vi "DMM Read DC Voltage.vi"() -> ()   [LabVIEW 2011]
uses:
  <instrlib>/DMM4/DMM4.lvlib
panel:
  out "error out":errorcluster
  out "Measure Value":string
  in  "Stop":bool
  out "Boolean":bool
  in  "Detector Rate":u16(ring) items=["SLOW", "MID", "FAST"]
  in  "Manual Range":dbl format="%#.9e"
  in  "Enable Auto Range":bool=TRUE
  out "ID Return String":string
  in  "Configure RS232 Baud Rate":u32(ring)=115200 items=["9600"=9600, "19200"=19200, "38400"=38400, "57600"=57600, "115200"=115200]
  in  "VISA resource name":refnum<visa-resource-name>
  # "DMM Read DC Voltage"
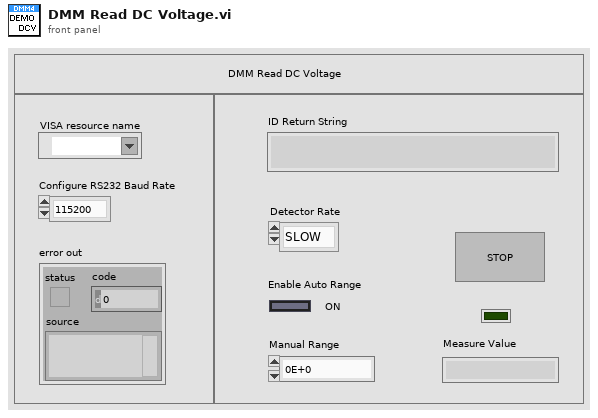
[diagram p1: front panel]
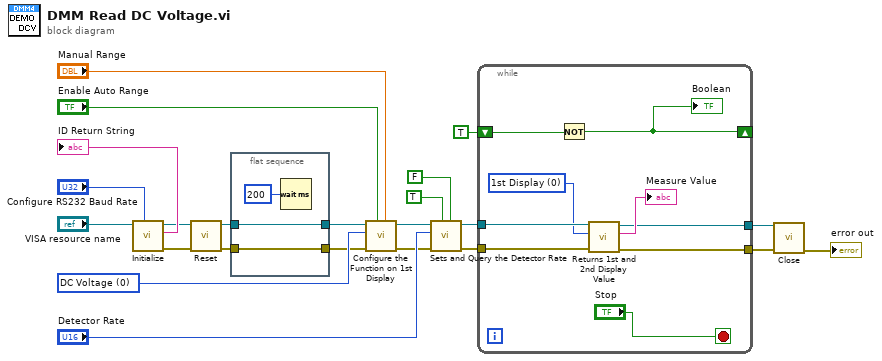
[diagram p0: block diagram]
diagram:
  w20 = u8 0 items=["DC Voltage", "AC Voltage", "DC+AC Voltage", "DC Current", "AC Current", "DC+AC Current", "2-Wire Resistance", "Frequency", "Period", "Continuity", "Diode", "Temperature", "Capacitance"] ("Function")
  n1 = call <instrlib>:"Initialize.vi"("Configure RS232 Baud Rate"="Configure RS232 Baud Rate", "VISA resource name"="VISA resource name") -> ("error out"=w6:errorcluster, "ID Return String"=→"ID Return String":string, "VISA resource name out"=w7:refnum<visa-resource-name>)  [unwired: 6 in, 1 out]
  n2 = call <instrlib>:"Reset.vi"("error in (no error)"=w6, "VISA resource name"=w7) -> ("error out"=w2:errorcluster, "VISA resource name out"=w4:refnum<visa-resource-name>)  [unwired: 8 in]
  n3 = flat-sequence {
    tunnel: w4 -> [w26]
    tunnel: [w26] -> w3
    tunnel: w2 -> [w25]
    tunnel: [w25] -> w1
    frame #0 {
      n4 = Wait (ms)(milliseconds to wait=u32 200) -> ()  [unwired: 1 out]
    }
  }
  n5 = call <instrlib>:"Configure the Function on 1st Display .vi"("Manual Range"="Manual Range", "Enable Auto Range"="Enable Auto Range", "error in"=w1, "Function"=w20, "VISA resource name"=w3) -> ("error out"=w8:errorcluster, "VISA resource name out"=w9:refnum<visa-resource-name>)  [unwired: 5 in]
  n6 = call <instrlib>:"Sets and Query the Detector Rate.vi"("Enable to Query"=FALSE, "Enable to Sets"=TRUE, "error in"=w8, "Detector Rate"="Detector Rate", "VISA resource name"=w9) -> ("error out"=w13:errorcluster, "VISA resource name out"=w14:refnum<visa-resource-name>)  [unwired: 4 in, 1 out]
  n7 = while {
    tunnel: w14 -> [w35]
    tunnel: w13 -> [w34]
    tunnel: [w30] -> w12
    tunnel: [w29] -> w11
    shift-right: [w27] -> _
    shift-left: TRUE -> [w28]
    stop <- "Stop" stop-if-true
    w33 = u16 0 items=["1st Display", "2nd Display", "1st & 2nd Display"] ("Sets to Display")
    n8 = Not(x=w28) -> (.not. x?=w27:bool)
    "Boolean" <- w27
    n9 = call <instrlib>:"Returns 1st and 2nd Display Value.vi"("error in"=w34, "Sets to Display"=w33, "VISA resource name"=w35) -> ("error out"=w29:errorcluster, "Return the Value"=→"Measure Value":string, "VISA resource name out"=w30:refnum<visa-resource-name>)  [unwired: 6 in]
  }
  n10 = call <instrlib>:"Close.vi"("error in (no error)"=w11, "VISA resource name"=w12) -> ("error out"=→"error out":errorcluster)  [unwired: 9 in]
